vi "GUI Step to RT Step.vi"(0 "GUI Step":T3) -> (4 "STEP":T1={"Direction"=enum."Chamber", "Pressure MPa"=0.0, "Time s"=0.0, "Delta alarm MPa"=0.0, "Delta warning MPa"=0.0})   [LabVIEW 2019]
uses:
  TypeDef/GUI Step.ctl
  TypeDef/Step.ctl
  TypeDef/Direction.ctl
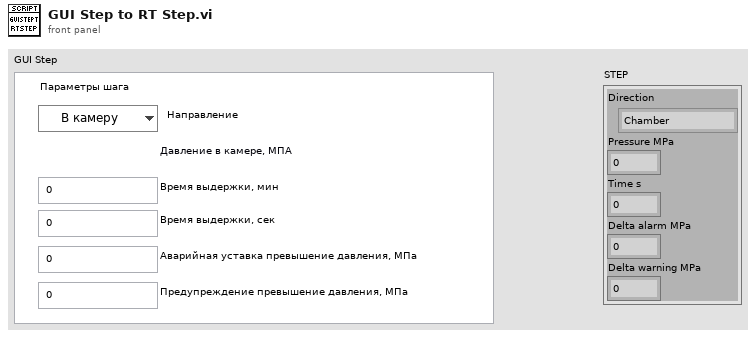
[diagram p1: front panel]
types:
  T1 = typedef "Step.ctl" = cluster{"Direction":T2, "Pressure MPa":dbl, "Time s":dbl, "Delta alarm MPa":dbl, "Delta warning MPa":dbl}
  T2 = typedef "Direction.ctl" = enum16{"None", "Chamber", "DUT"}
  T3 = typedef "GUI Step.ctl" = cluster{"pressure MPa":dbl, "time min":dbl, "delta alarm MPa":dbl, "direction":enum16{"В камеру", "В образец"}, "delta warning MPa":dbl, "time sec":dbl}
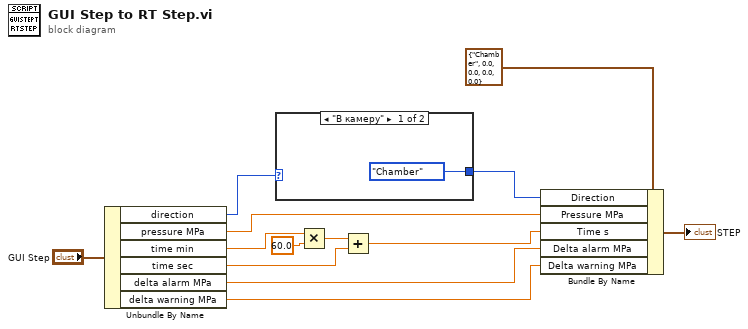
[diagram p0: block diagram]
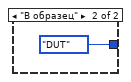
[diagram p2: hidden frame]
diagram:
  n1 = Unbundle By Name("GUI Step") -> ("direction"=w10:enum16{"В камеру", "В образец"}, "pressure MPa"=w8:dbl, "time min"=w7:dbl, "time sec"=w4:dbl, "delta alarm MPa"=w2:dbl, "delta warning MPa"=w1:dbl)
  n2 = case shown="\"В камеру\"" w10 {
    tunnel: [Direction."Chamber" ("Direction") Direction."DUT" ("Direction")] -> w9
    frame "В камеру" {
    }
    frame "В образец" {
    }
  }
  n3 = Multiply(x=w7, y=60.0) -> (x*y=w5:dbl)
  n4 = Add(x=w5, y=w4) -> (x+y=w3:dbl)
  n5 = Bundle By Name(cluster=T1 {"Direction"=enum."Chamber", "Pressure MPa"=0.0, "Time s"=0.0, "Delta alarm MPa"=0.0, "Delta warning MPa"=0.0} ("STEP"), "Direction"=w9, "Pressure MPa"=w8, "Time s"=w3, "Delta alarm MPa"=w2, "Delta warning MPa"=w1) -> (→"STEP":T1)
